vi "GPS -Evnt Mouse DblClick.vi"(4 "output cluster":T1, 5 "Event Data":cluster{"sender":refnum<k24>, "e":refnum<k24>}, 6 "Control Ref":refnum<k24>, 7 "Event Common Data":T2) -> ()   [LabVIEW 2019]
uses:
  \\mac\Dropbox/gmap.net/GMAP.NET 8.6/data/GMap.NET.WindowsForms.dll
  data/GMap.NET.WindowsForms.dll
  System.Windows.Forms
  ctlSeqFNs -GPSLocation.ctl
  ctlInput4PtsColl.ctl
  \\mac\Dropbox/gmap.net/GMAP.NET 8.6/data/GMap.NET.Core.dll
  data/GMap.NET.Core.dll
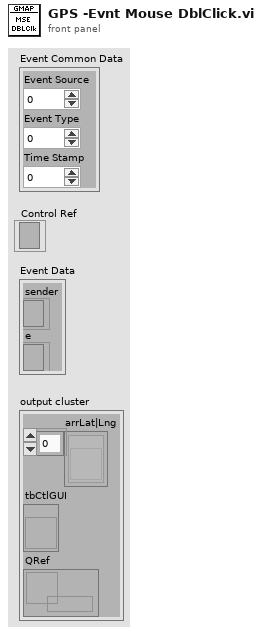
[diagram p1: front panel]
types:
  T1 = cluster{"arrLat|Lng":refnum<vi>[], "tbCtlGUI":refnum<vi>, "QRef":refnum<queue>}
  T2 = cluster{"Event Source":i32, "Event Type":u32, "Time Stamp":u32}
  T3 = typedef "ctlSeqFNs -GPSLocation.ctl" = enum16{"pre-init", "preinit01", "preinit02", "preinit03", "preinit04", "preinit05", "init", "idle", "GUI -Pop Menu", "GUI -Add Marker Combo", "GUI -Annotate Grid", "ALIGN COLS", "SET -Provider", "SET -SCALE", "OVERLAY -ADD", "POINTS -CREATE LIST (Container)", "MARKERS -CREATE LIST", "MAP -MARKER Add Or Rmv", "DOWNLOAD -Project Addr", "MAP -Marker Update", "MAP -Save", "MAP -Markers Autofit", "MAP -Addr to Lat + Lng", "MAP -Markers Clear", "PIN DROP -Get Nearest", "AUDIT -Use Marker Shown", "error", "exit"}
  T4 = typedef "ctlInput4PtsColl.ctl" = cluster{"arrLatLngActv":dbl[][], "ptKeyorID":string[], "Add":bool}
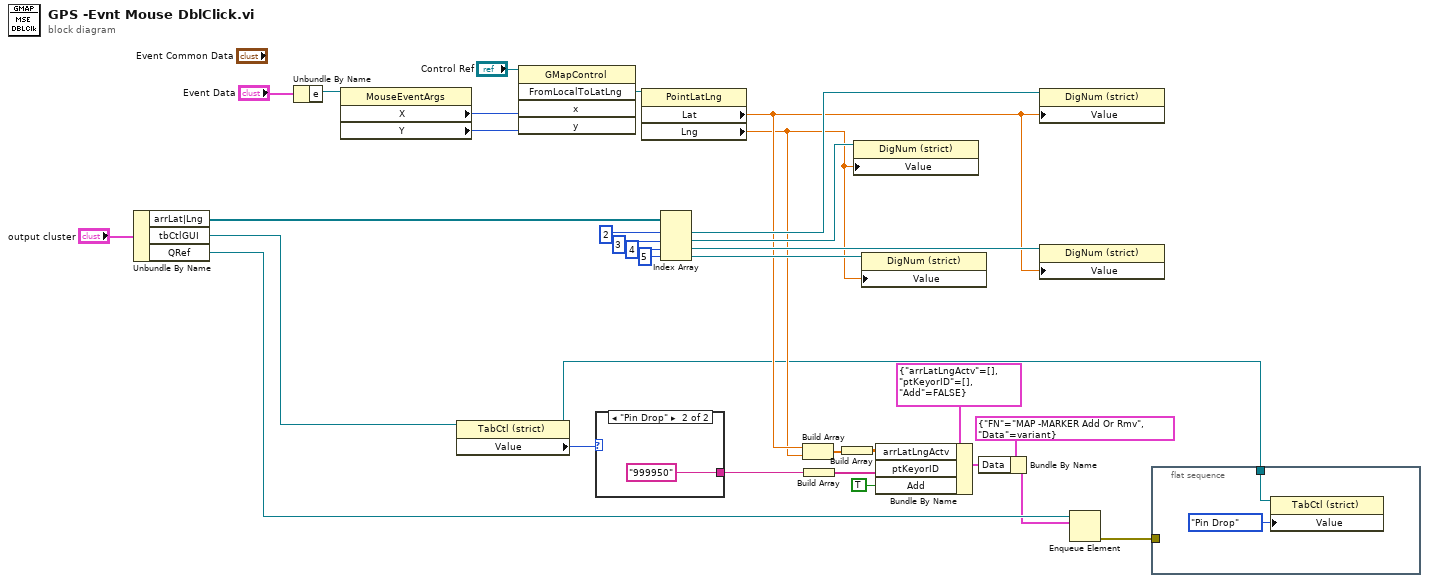
[diagram p0: block diagram]
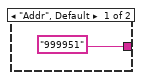
[diagram p2: hidden frame]
diagram:
  n1 = Unbundle By Name("output cluster") -> ("arrLat|Lng"=w17:refnum<vi>[], "tbCtlGUI"=w16:refnum<vi>, "QRef"=w15:refnum<queue>)
  n2 = Unbundle By Name("Event Data") -> ("e"=w29:refnum<k24>)
  n3 = property class="MouseEventArgs"(reference=w29) -> ("X"=w28:i32, "Y"=w27:i32)  [unwired: 1 in, 2 out]
  n4 = property class="TabCtl (strict)"(reference=w16) -> (reference out=w1:refnum<vi>, "Value"=w7:enum32{"Position", "Pin Drop", "Addr", "Setup"})  [unwired: 1 in, 1 out]
  n5 = invoke class="GMapControl" method="FromLocalToLatLng"(reference="Control Ref", "x"=w28, "y"=w27) -> ("FromLocalToLatLng"=w31:refnum<k24>)  [unwired: 2 in, 4 out]
  n6 = case shown="\"Pin Drop\"" w7 {
    tunnel: ["999951" "999950"] -> w9
    frame "Addr", Default {
    }
    frame "Pin Drop" {
    }
  }
  n7 = property class="PointLatLng"(reference=w31) -> ("Lat"=w14:dbl, "Lng"=w13:dbl)  [unwired: 1 in, 2 out]
  n8 = Index Array(array=w17, index #1=2 ("index"), index #2=3 ("index"), index #3=4 ("index"), index #4=5 ("index")) -> (element #1=w25:refnum<vi>, element #2=w24:refnum<vi>, element #3=w23:refnum<vi>, element #4=w22:refnum<vi>)
  n9 = Build Array(w14, w13) -> (w11:dbl[])
  n10 = Build Array(w9) -> (w8:string[])
  n11 = Build Array(w11) -> (w10:dbl[][])
  n12 = property class="DigNum (strict)"(reference=w24, "Value"=w13) -> ()  [unwired: 1 in, 2 out]
  n13 = property class="DigNum (strict)"(reference=w22, "Value"=w13) -> ()  [unwired: 1 in, 2 out]
  n14 = Bundle By Name(cluster=T4 {"arrLatLngActv"=[], "ptKeyorID"=[], "Add"=FALSE} ("PtLatLn+KywrdOrID"), "arrLatLngActv"=w10, "ptKeyorID"=w8, "Add"=TRUE) -> (w5:T4)
  n15 = Bundle By Name(cluster=cluster{"FN":T3, "Data":variant} {"FN"=enum."MAP -MARKER Add Or Rmv", "Data"=variant} ("element"), "Data"=w5) -> (w4:cluster{"FN":T3, "Data":variant})
  n16 = property class="DigNum (strict)"(reference=w25, "Value"=w14) -> ()  [unwired: 1 in, 2 out]
  n17 = property class="DigNum (strict)"(reference=w23, "Value"=w14) -> ()  [unwired: 1 in, 2 out]
  n18 = Enqueue Element(queue=w15, element=w4) -> (error out=w2:errorcluster)  [unwired: 2 in, 2 out]
  n19 = flat-sequence {
    tunnel: w2 -> [_]
    tunnel: w1 -> [w36]
    frame #0 {
      n20 = property class="TabCtl (strict)"(reference=w36, "Value"=enum32{"Position", "Pin Drop", "Addr", "Setup"}."Pin Drop") -> ()  [unwired: 1 in, 2 out]
    }
  }
